vi "Write Data to File.vi"(8 "error in":errorcluster, 11 "tCRD in":refnum<class "Aircraft OPCCRD.lvclass">) -> (0 "error out":errorcluster, 3 "tCRD out":refnum<class "Aircraft OPCCRD.lvclass">)   [LabVIEW 2015, in "Aircraft OPCCRD.lvclass"]
uses:
  Aircraft OPCCRD.lvclass
  Data/tCRD Data.lvclass
  Reusable/Data/Data.lvclass
  Aircraft OPCCRD.lvclass/Aircraft OPCCRD.ctl
  Reusable/CRDS/Main/CRDS.lvclass/CRDS.ctl
  Reusable/Observer/Data Subject.lvclass/Data Subject.ctl
  Reusable/File IO/Class/File Observer.lvclass/File Observer.ctl
  Reusable/CRDS/Data/Cell/CRDS Cell Data.lvclass/CRDS Cell Data.ctl
  Data/tCRD Data.lvclass/tCRD Data.ctl
  Reusable/CRDS/Data/Cell/Read extParam.vi
  Reusable/CRDS/Data/Cell/Write extParam.vi
  Accessors/Read CRD Subj.vi
  Reusable/CRDS/Main/Read Laser Data.vi
  Reusable/Observer/Accessors/Read Observer Refs.vi
  Reusable/Observer/Accessors/Read DVR.vi
  Data/Accessors/Write file path.vi
  Data/Accessors/Write file size.vi
  Reusable/CRDS/Main/Read Data.vi
  Reusable/CRDS/Data/Main/Write CellData.vi
  Reusable/CRDS/Data/Main/CRDS Data.lvclass
  Data Subj/tCRDS Subj.lvclass
  Reusable/Instrument/Instrument.lvclass
  Reusable/CRDS/Data/Cell/CRDS Cell Data.lvclass
  Reusable/File IO/Class/File Observer.lvclass
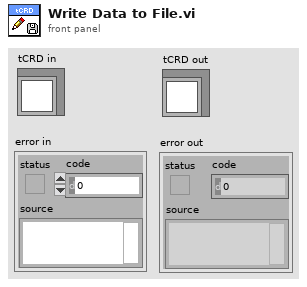
[diagram p1: front panel]
types:
  T1 = typedef "extparam.ctl" = cluster{"Tau":sgl, "Tau0cor":sgl, "ext":sgl, "extCorr":sgl, "stdevTau":sgl, "eTau":sgl, "taucorr":sgl, "Tau0":sgl, "max":sgl}
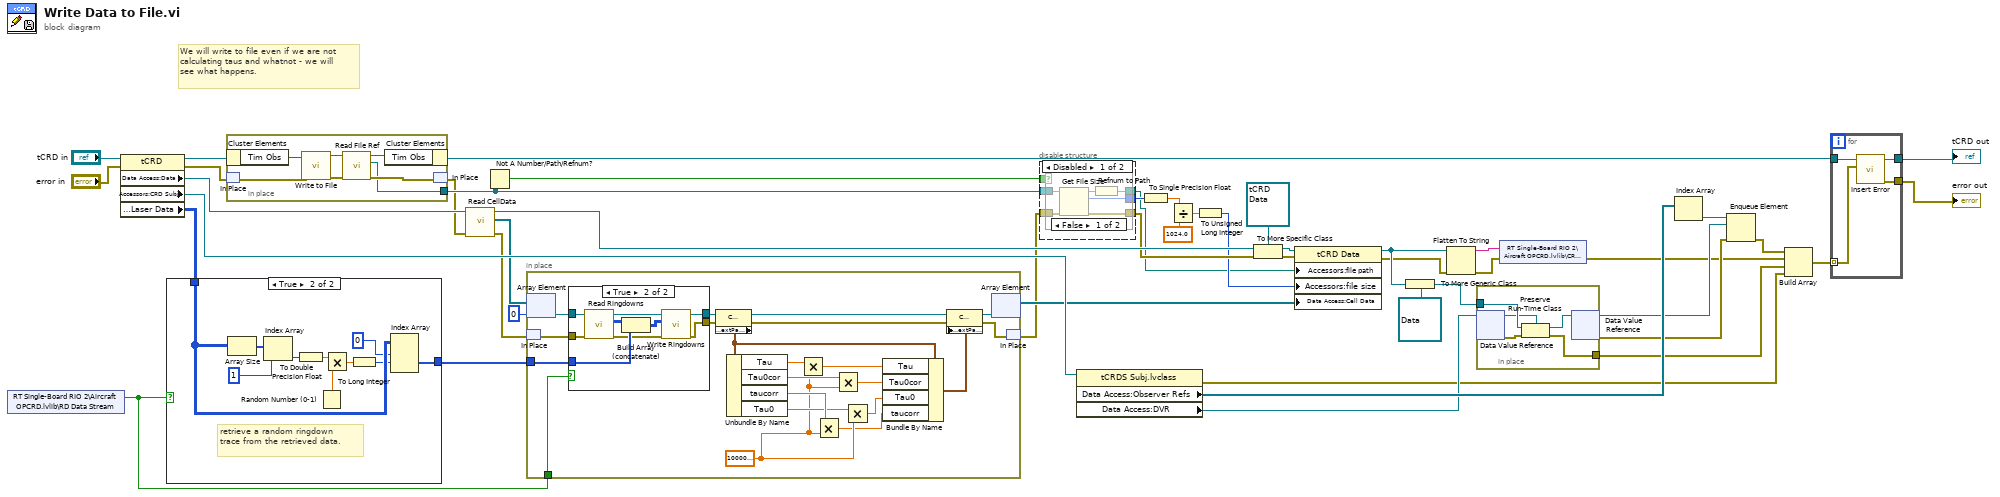
[diagram p0: block diagram]
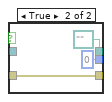
[diagram p4: hidden frame]
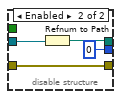
[diagram p5: hidden frame]
diagram:
  # "We will write to file even if we are not calculating taus and whatnot - we will see what happens."
  n1 = shared-variable "RT Single-Board RIO 2\\Aircraft OPCRD.lvlib\\RD Data Stream"() -> (w1:bool)  [unwired: 1 in, 1 out]
  n2 = property class="tCRD"(reference="tCRD in", error in="error in") -> (reference out=w41:refnum<class "Aircraft OPCCRD.lvclass">, error out=w40:errorcluster, "Data Access:Data"=w37:refnum<class "CRDS Data.lvclass">, "Accessors:CRD Subj"=w43:refnum<class "tCRDS Subj.lvclass">, "Data Access:Laser Data"=w42:i16[][][])
  n3 = case shown="True" w1 {
    tunnel: w42 -> [_ w57]
    tunnel: [_ w56] -> w6
    frame False {
    }
    frame True {
      # "retrieve a random ringdown trace from the retrieved data."
      n4 = Array Size(array=w57) -> (size(s)=w53:i32[])
      n5 = Index Array(array=w53, index=1) -> (element=w52:i32)
      n6 = To Double Precision Float(number=w52) -> (double precision float=w51:dbl)
      n7 = Random Number (0-1)() -> (number: 0 to 1=w55:dbl)
      n8 = Multiply(x=w51, y=w55) -> (x*y=w54:dbl)
      n9 = To Long Integer(number=w54) -> (32bit integer=w48:i32)
      n10 = Index Array(array=w57, index (dim 0)=0 ("index (page)"), index (dim 1)=w48) -> (element=w56:i16[])  [unwired: 1 in]
    }
  }
  n11 = in-place {
    in-place-border: [w62] -> w39
    n12 = in-place-cluster #1(w41) -> ("Tim Obs"=w61:refnum<class "Tim File Observer.lvclass">)
    n13 = in-place-match #2(w40) -> (w59:errorcluster)
    n14 = call "Write to File.vi"("error in"=w59, "File Obs in"=w61) -> ("error out"=w58:errorcluster, "File Obs out"=w60:refnum<class "Tim File Observer.lvclass">)  [unwired: 8 in]
    n15 = call "Read File Ref.vi"("error in"=w58, "File Observer in"=w60) -> ("error out"=w63:errorcluster, "File Ref"=w62:refnum<file>, "File Observer out"=w64:refnum<class "Tim File Observer.lvclass">)  [unwired: 7 in]
    n16 = in-place-cluster #1("Tim Obs"=w64) -> (w38:refnum<class "Aircraft OPCCRD.lvclass">)
    n17 = in-place-match #2(w63) -> (w34:errorcluster)
  }
  n18 = call "Read CellData.vi"("error in"=w34, "CRDS Data in"=w37) -> ("error out"=w33:errorcluster, "CellData"=w36:refnum<class "CRDS Cell Data.lvclass">[], "CRDS Data out"=w35:refnum<class "CRDS Data.lvclass">)  [unwired: 7 in]
  n19 = Not A Number/Path/Refnum?(number/path/refnum=w39) -> (NaN/Path/Refnum?=w17:bool)
  n20 = in-place {
    in-place-border: w6 -> [w85]
    in-place-border: w1 -> [w65]
    w72 = sgl 1000000.0 ("y")
    n21 = in-place-array #3(w36, 0) -> (w84:refnum<class "CRDS Cell Data.lvclass">)
    n22 = in-place-match #4(w33) -> (w83:errorcluster)
    n23 = case shown="True" w65 {
      tunnel: w85 -> [_ w96]
      tunnel: w84 -> [w87 w95]
      tunnel: w83 -> [w86 w90]
      tunnel: [w87 w89] -> w82
      tunnel: [w86 w88] -> w80
      frame False {
      }
      frame True {
        n24 = call "Read Ringdowns.vi"("error in (no error)"=w90, "CRDS Cell Data in"=w95) -> ("error out"=w92:errorcluster, "Ringdowns"=w94:i16[][], "CRDS Cell Data out"=w93:refnum<class "CRDS Cell Data.lvclass">)  [unwired: 7 in]
        n25 = Build Array (concatenate)(w94, w96) -> (w91:i16[][])
        n26 = call "Write Ringdowns.vi"("error in"=w92, "Ringdowns"=w91, "CRDS Cell Data in"=w93) -> ("error out"=w88:errorcluster, "CRDS Cell Data out"=w89:refnum<class "CRDS Cell Data.lvclass">)  [unwired: 7 in]
      }
    }
    n27 = property class="CRDS Cell"(reference=w82, error in=w80) -> (reference out=w78:refnum<class "CRDS Cell Data.lvclass">, error out=w79:errorcluster, "Data Access:extParam"=w71:T1)
    n28 = Unbundle By Name(w71) -> ("Tau"=w76:sgl, "Tau0cor"=w75:sgl, "taucorr"=w74:sgl, "Tau0"=w73:sgl)
    n29 = Multiply(x=w76, y=w72) -> (x*y=w69:sgl)
    n30 = Multiply(x=w74, y=w72) -> (x*y=w66:sgl)
    n31 = Multiply(x=w75, y=w72) -> (x*y=w68:sgl)
    n32 = Multiply(x=w73, y=w72) -> (x*y=w67:sgl)
    n33 = Bundle By Name(cluster=w71, "Tau"=w69, "Tau0cor"=w68, "Tau0"=w67, "taucorr"=w66) -> (w70:T1)
    n34 = property class="CRDS Cell"(reference=w78, error in=w79, "Data Access:extParam"=w70) -> (reference out=w81:refnum<class "CRDS Cell Data.lvclass">, error out=w77:errorcluster)
    n35 = in-place-array #3(w81) -> (w21:refnum<class "CRDS Cell Data.lvclass">[])  [unwired: 1 out]
    n36 = in-place-match #4(w77) -> (w20:errorcluster)
  }
  n37 = disable-structure shown="Disabled" {
    disable-tunnel: w39 -> [w102 w114]
    disable-tunnel: [w101 w115] -> w22
    disable-tunnel: [w100 w113] -> w7
    disable-tunnel: w20 -> [w99 w115]
    disable-tunnel: w17 -> [w98 _]
    disable-tunnel: [w97 i64 0 ("size (in bytes)")] -> w11
    frame Disabled {
      n38 = case shown="False" w98 {
        tunnel: [w108 w109] -> w101
        tunnel: [w107 i64 0 ("size (in bytes)")] -> w97
        tunnel: [w105 path ""] -> w100
        tunnel: w102 -> [w104 _]
        tunnel: w99 -> [w103 w109]
        frame False {
          n39 = Get File Size(file=w104, error in=w103) -> (refnum out=w106:refnum<file>, size (in bytes)=w107:i64, 0:w108:errorcluster)
          n40 = Refnum to Path(1:w106) -> (0:w105:path)
        }
        frame True {
        }
      }
    }
    frame Enabled {
      n41 = Refnum to Path(1:w114) -> (0:w113:path)
    }
  }
  n42 = property class="tCRDS Subj.lvclass"(reference=w43) -> (error out=w26:errorcluster, "Data Access:Observer Refs"=w32:refnum<queue>[], "Data Access:DVR"=w30:refnum<data-value>)  [unwired: 1 in, 1 out]
  n43 = To Single Precision Float(number=w11) -> (single precision float=w10:sgl)
  n44 = Divide(x=w10, y=sgl 1024.0) -> (x/y=w9:sgl)
  n45 = To Unsigned Long Integer(number=w9) -> (unsigned 32bit integer=w13:u32)
  n46 = To More Specific Class(target class=refnum<class "tCRD Data.lvclass"> refnum ("tCRD Data"), reference=w35, error in=w22) -> (specific class reference=w24:refnum<class "tCRD Data.lvclass">, error out=w23:errorcluster)
  n47 = property class="tCRD Data"(reference=w24, error in=w23, "Accessors:file path"=w7, "Accessors:file size"=w13, "Data Access:Cell Data"=w21) -> (reference out=w15:refnum<class "tCRD Data.lvclass">, error out=w14:errorcluster)
  n48 = To More Generic Class(target class=refnum<class "Data.lvclass"> refnum ("Base Data Class.lvlib:Data"), reference=w15) -> (generic class reference=w31:refnum<class "Data.lvclass">)
  n49 = Flatten To String(anything=w15, error in (no error)=w14) -> (data string=w4:string, error out=w3:errorcluster)  [unwired: 2 in, 1 out]
  n50 = in-place {
    in-place-border: w31 -> [w120]
    in-place-border: [w116] -> w27
    n51 = in-place-dvr #5(w30) -> (w119:refnum<class "Data.lvclass">, w117:errorcluster)
    n52 = Preserve Run-Time Class(object in=w120, error in=w117, 2:w119) -> (object out=w118:refnum<class "Data.lvclass">, error out=w116:errorcluster)
    n53 = in-place-dvr #5(w118) -> (w29:refnum<data-value>, w28:errorcluster)
  }
  n54 = shared-variable "RT Single-Board RIO 2\\Aircraft OPCRD.lvlib\\CRD Data"(w4, error in=w3) -> (error out=w19:errorcluster)
  n55 = Index Array(array=w32) -> (element=w2:refnum<queue>)  [unwired: 1 in]
  n56 = Enqueue Element(queue=w2, element=w29, error in (no error)=w28) -> (error out=w18:errorcluster)  [unwired: 1 in, 2 out]
  n57 = Build Array(w18, w19, w27, w26) -> (w44:errorcluster[])
  n58 = for {
    tunnel: w44 -> [w122] mode=indexing
    tunnel: w38 -> [w124]
    tunnel: [w123] -> w47
    tunnel: [w121] -> w46
    n59 = call "Insert Error.vi"("err"=w122, "Instrument in"=w124) -> ("error out"=w121:errorcluster, "Instrument out"=w123:refnum<class "Aircraft OPCCRD.lvclass">)  [unwired: 7 in, 1 out]
  }
  "error out" <- w46
  "tCRD out" <- w47
